vi "Write Enabled_.vi"(8 "error in (no error)":errorcluster, 10 "Enabled?":bool[](array[boolean]), 11 "Lesker Pressure in":refnum<class "Lesker Pressure.lvclass">) -> (0 "error out":errorcluster, 3 "Lesker Pressure out":refnum<class "Lesker Pressure.lvclass">)   [LabVIEW 2021, in "Lesker Pressure.lvclass"]
uses:
  Lesker Pressure.lvclass
  Lesker Pressure.lvclass/Lesker Pressure.ctl
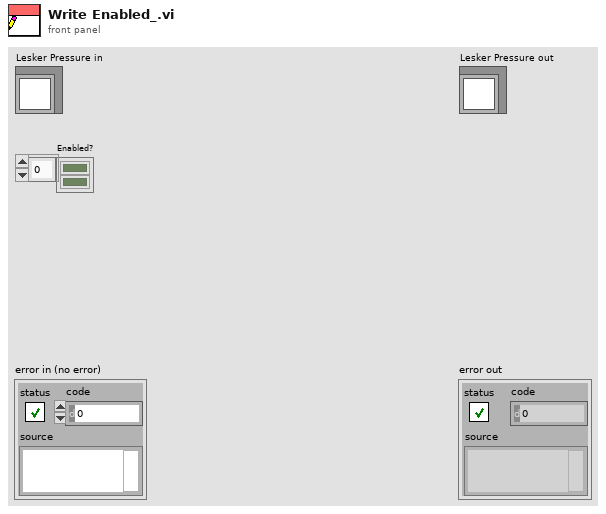
[diagram p1: front panel]
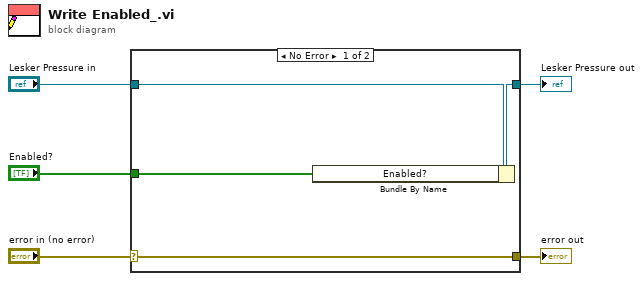
[diagram p0: block diagram]
diagram:
  n1 = case shown="No Error" "error in (no error)" {
    selector: "error in (no error)" -> [w9 w10]
    tunnel: [w9 w10] -> w4
    tunnel: [w7 w11] -> w2
    tunnel: "Lesker Pressure in" -> [w8 w11]
    tunnel: "Enabled?" -> [w6 _]
    frame No Error {
      n2 = Bundle By Name(cluster=w8, "Enabled?"=w6) -> (w7:refnum<class "Lesker Pressure.lvclass">)
    }
    frame Error {
    }
  }
  "error out" <- w4
  "Lesker Pressure out" <- w2
